vi "5-Lissajous Figures.vi"() -> ()   [LabVIEW 2020]
panel:
  out "XY Graph":cluster{dbl[], dbl[]}(graph)
  in  "Knob":dbl(knob) scale=0.0..180.0
  in  "stop":bool
  in  "a2":dbl=1.0
  in  "a1":dbl=1.0
  # "User can switch among figures\nby changing the control values."
  # "Knob is incremented by loop\niteration to turn the figure automatically."
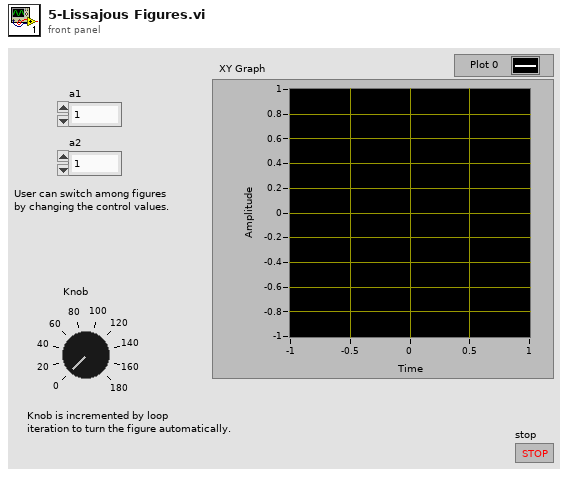
[diagram p1: front panel]
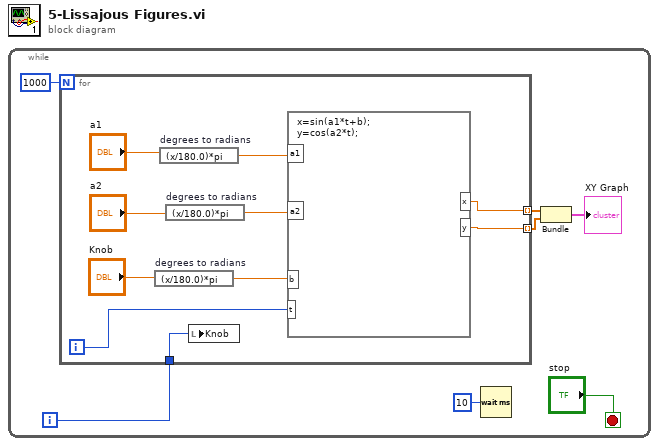
[diagram p0: block diagram]
diagram:
  n1 = while {
    i -> [w1]
    stop <- "stop" stop-if-true
    n2 = for {
      N: 1000 -> [_]
      tunnel: [w11] -> w5 mode=indexing
      tunnel: [w10] -> w4 mode=indexing
      tunnel: w1 -> [w8]
      i -> [w9]
      n3 = expression code="(x/180.0)*pi" "degrees to radians"("Knob") -> (w17:dbl)
      n4 = expression code="(x/180.0)*pi" "degrees to radians"("a1") -> (w15:dbl)
      n5 = expression code="(x/180.0)*pi" "degrees to radians"("a2") -> (w13:dbl)
      n6 = local write "Knob"(w8) -> ()
      n7 = formula code="x=sin(a1*t+b);\ny=cos(a2*t);"("a1"=w15, "a2"=w13, "b"=w17, "t"=w9) -> ("x"=w11:dbl, "y"=w10:dbl)
    }
    n8 = Wait (ms)(milliseconds to wait=u32 10) -> ()  [unwired: 1 out]
    n9 = Bundle(w5, w4) -> (→"XY Graph":cluster{dbl[], dbl[]})  [unwired: 1 in]
  }
